vi "Vacuum On.vi"() -> (0 "error out":errorcluster)   [LabVIEW 2025]
doc: "Turns on the vacuum table to hold the UUT in place on the test fixture."
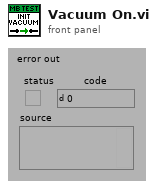
[diagram p1: front panel]
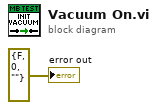
[diagram p0: block diagram]
diagram:
  "error out" <- errorcluster {"status"=FALSE, "code"=0, "source"=""} ("error out")
